vi "Using GXML For Packet Data Description.vi"() -> ()   [LabVIEW 2014]
uses:
  <vilib>/NI/GXML/_subVIs/GXML SearchParser/Search Parser.vi
  <vilib>/NI/GXML/GXML.lvlib
panel:
  out "data":T1(array[cluster])
  out "error out":errorcluster
  out "XML String Out":string
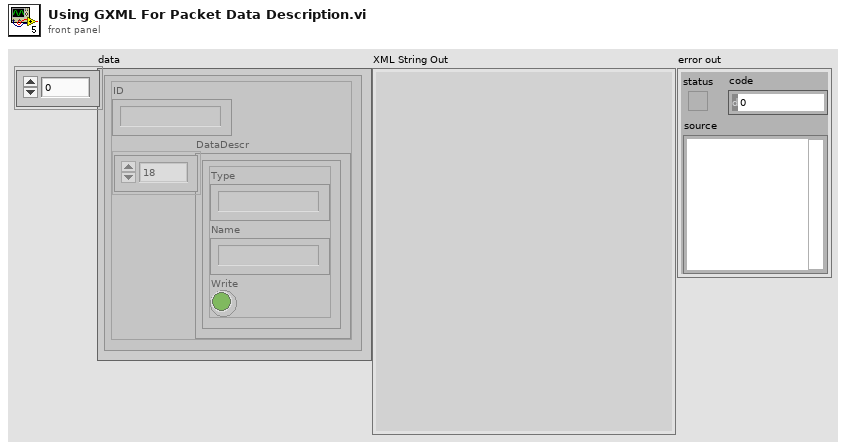
[diagram p1: front panel]
types:
  T1 = cluster{"ID":string, "DataDescr":cluster{"Type":string, "Name":string, "Write":bool}[]}[]
  T2 = cluster{"ID":string, "DataDescr":cluster{"Type":string, "Name":string, "Var":string, "Write":bool}[]}[]
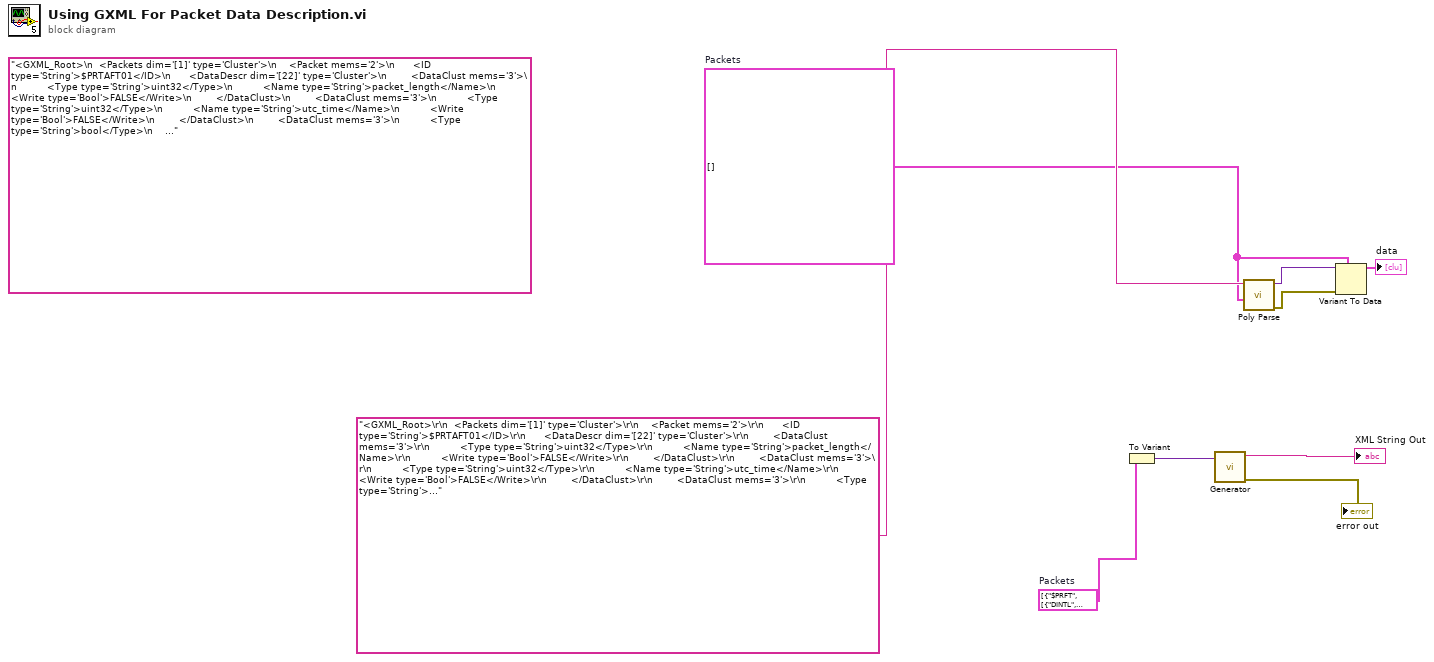
[diagram p0: block diagram]
diagram:
  w1 = T1 []  # Packets
  (unwired) "<GXML_Root>\n  <Packets dim='[1]' type='Cluster'>\n    <Packet mems='2'>\n      <ID type='String'>$PRTAFT01</ID>\n      <DataDescr dim='[22]' type='Cluster'>\n        <DataClust mems='3'>\n          <Type type='String'>uint32</Type>\n          <Name type='String'>packet_length</Name>\n          <Write type='Bool'>FALSE</Write>\n        </DataClust>\n        <DataClust mems='3'>\n          <Type type='String'>uint32</Type>\n          <Name type='String'>utc_time</Name>\n          <Write type='Bool'>FALSE</Write>\n        </DataClust>\n        <DataClust mems='3'>\n          <Type type='String'>bool</Type>\n          <Name type='String'>ptp_sync</Name>\n          <Write type='Bool'>FALSE</Write>\n        </DataClust>\n        <DataClust mems='3'>\n          <Type type='String'>uint32</Type>\n          <Name type='String'>crio_temp</Name>\n          <Write type='Bool'>FALSE</Write>\n        </DataClust>\n        <DataClust mems='3'>\n          <Type type='String'>str</Type>\n          <Name type='String'>flight_num</Name>\n          <Write type='Bool'>FALSE</Write>\n        </DataClust>\n        <DataClust mems='3'>\n          <Type type='String'>uint8</Type>\n          <Name type='String'>crio_fpga_run</Name>\n          <Write type='Bool'>FALSE</Write>\n        </DataClust>\n        <DataClust mems='3'>\n          <Type type='String'>uint8</Type>\n          <Name type='String'>crio_rtc_run</Name>\n          <Write type='Bool'>FALSE</Write>\n        </DataClust>\n        <DataClust mems='3'>\n          <Type type='String'>uint8</Type>\n          <Name type='String'>crio_status</Name>\n          <Write type='Bool'>FALSE</Write>\n        </DataClust>\n        <DataClust mems='3'>\n          <Type type='String'>uint16</Type>\n          <Name type='String'>crio_UDP_num</Name>\n          <Write type='Bool'>FALSE</Write>\n        </DataClust>\n        <DataClust mems='3'>\n          <Type type='String'>str</Type>\n          <Name type='String'>crio_mem_used</Name>\n          <Write type='Bool'>FALSE</Write>\n        </DataClust>\n        <DataClust mems='3'>\n          <Type type='String'>str</Type>\n          <Name type='String'>crio_disktype</Name>\n          <Write type='Bool'>FALSE</Write>\n        </DataClust>\n        <DataClust mems='3'>\n          <Type type='String'>str</Type>\n          <Name type='String'>crio_aux_out3</Name>\n          <Write type='Bool'>FALSE</Write>\n        </DataClust>\n        <DataClust mems='3'>\n          <Type type='String'>uint32</Type>\n          <Name type='String'>pressure_alt</Name>\n          <Write type='Bool'>FALSE</Write>\n        </DataClust>\n        <DataClust mems='3'>\n          <Type type='String'>int32</Type>\n          <Name type='String'>ind_air_speed</Name>\n          <Write type='Bool'>FALSE</Write>\n        </DataClust>\n        <DataClust mems='3'>\n          <Type type='String'>int32</Type>\n          <Name type='String'>rad_alt</Name>\n          <Write type='Bool'>FALSE</Write>\n        </DataClust>\n        <DataClust mems='3'>\n          <Type type='String'>uint8</Type>\n          <Name type='String'>unused_1</Name>\n          <Write type='Bool'>FALSE</Write>\n        </DataClust>\n        <DataClust mems='3'>\n          <Type type='String'>uint8</Type>\n          <Name type='String'>unused_2</Name>\n          <Write type='Bool'>FALSE</Write>\n        </DataClust>\n        <DataClust mems='3'>\n          <Type type='String'>uint8</Type>\n          <Name type='String'>deiced_temp_flag</Name>\n          <Write type='Bool'>FALSE</Write>\n        </DataClust>\n        <DataClust mems='3'>\n          <Type type='String'>uint8</Type>\n          <Name type='String'>wow_flag</Name>\n          <Write type='Bool'>FALSE</Write>\n        </DataClust>\n        <DataClust mems='3'>\n          <Type type='String'>uint8</Type>\n          <Name type='String'>heimann_calib_flag</Name>\n          <Write type='Bool'>FALSE</Write>\n        </DataClust>\n        <DataClust mems='3'>\n          <Type type='String'>int32</Type>\n          <Name type='String'>jci140_signal</Name>\n          <Write type='Bool'>FALSE</Write>\n        </DataClust>\n        <DataClust mems='3'>\n          <Type type='String'>int32</Type>\n          <Name type='String'>jci140_range</Name>\n          <Write type='Bool'>FALSE</Write>\n        </DataClust>\n      </DataDescr>\n    </Packet>\n  </Packets>\n</GXML_Root>\n"
  w6 = T2 [{"ID"="$PRFT", "DataDescr"=[{"Type"="DINTL", "Name"="GenericInt 1", "Var"="crd_int", "Write"=TRUE}, {"Type"="DBL", "Name"="Generic DBL", "Var"="pas_dbl", "Write"=TRUE}]}]  # Packets
  n1 = To Variant(anything=w6) -> (Variant=w9:variant)
  n2 = call <vilib>:"Generator.vi"("Variant"=w9) -> ("error out"=→"error out":errorcluster, "XML String Out"=→"XML String Out":string)  [unwired: 9 in]
  n3 = call-poly <vilib>:"Poly Parse.vi"("TypeDesc"=w1, "XML String In"="<GXML_Root>\r\n  <Packets dim='[1]' type='Cluster'>\r\n    <Packet mems='2'>\r\n      <ID type='String'>$PRTAFT01</ID>\r\n      <DataDescr dim='[22]' type='Cluster'>\r\n        <DataClust mems='3'>\r\n          <Type type='String'>uint32</Type>\r\n          <Name type='String'>packet_length</Name>\r\n          <Write type='Bool'>FALSE</Write>\r\n        </DataClust>\r\n        <DataClust mems='3'>\r\n          <Type type='String'>uint32</Type>\r\n          <Name type='String'>utc_time</Name>\r\n          <Write type='Bool'>FALSE</Write>\r\n        </DataClust>\r\n        <DataClust mems='3'>\r\n          <Type type='String'>bool</Type>\r\n          <Name type='String'>ptp_sync</Name>\r\n          <Write type='Bool'>FALSE</Write>\r\n        </DataClust>\r\n        <DataClust mems='3'>\r\n          <Type type='String'>uint32</Type>\r\n          <Name type='String'>crio_temp</Name>\r\n          <Write type='Bool'>FALSE</Write>\r\n        </DataClust>\r\n        <DataClust mems='3'>\r\n          <Type type='String'>str</Type>\r\n          <Name type='String'>flight_num</Name>\r\n          <Write type='Bool'>FALSE</Write>\r\n        </DataClust>\r\n        <DataClust mems='3'>\r\n          <Type type='String'>uint8</Type>\r\n          <Name type='String'>crio_fpga_run</Name>\r\n          <Write type='Bool'>FALSE</Write>\r\n        </DataClust>\r\n        <DataClust mems='3'>\r\n          <Type type='String'>uint8</Type>\r\n          <Name type='String'>crio_rtc_run</Name>\r\n          <Write type='Bool'>FALSE</Write>\r\n        </DataClust>\r\n        <DataClust mems='3'>\r\n          <Type type='String'>uint8</Type>\r\n          <Name type='String'>crio_status</Name>\r\n          <Write type='Bool'>FALSE</Write>\r\n        </DataClust>\r\n        <DataClust mems='3'>\r\n          <Type type='String'>uint16</Type>\r\n          <Name type='String'>crio_UDP_num</Name>\r\n          <Write type='Bool'>FALSE</Write>\r\n        </DataClust>\r\n        <DataClust mems='3'>\r\n          <Type type='String'>str</Type>\r\n          <Name type='String'>crio_mem_used</Name>\r\n          <Write type='Bool'>FALSE</Write>\r\n        </DataClust>\r\n        <DataClust mems='3'>\r\n          <Type type='String'>str</Type>\r\n          <Name type='String'>crio_disktype</Name>\r\n          <Write type='Bool'>FALSE</Write>\r\n        </DataClust>\r\n        <DataClust mems='3'>\r\n          <Type type='String'>str</Type>\r\n          <Name type='String'>crio_aux_out3</Name>\r\n          <Write type='Bool'>FALSE</Write>\r\n        </DataClust>\r\n        <DataClust mems='3'>\r\n          <Type type='String'>uint32</Type>\r\n          <Name type='String'>pressure_alt</Name>\r\n          <Write type='Bool'>FALSE</Write>\r\n        </DataClust>\r\n        <DataClust mems='3'>\r\n          <Type type='String'>int32</Type>\r\n          <Name type='String'>ind_air_speed</Name>\r\n          <Write type='Bool'>FALSE</Write>\r\n        </DataClust>\r\n        <DataClust mems='3'>\r\n          <Type type='String'>int32</Type>\r\n          <Name type='String'>rad_alt</Name>\r\n          <Write type='Bool'>FALSE</Write>\r\n        </DataClust>\r\n        <DataClust mems='3'>\r\n          <Type type='String'>uint8</Type>\r\n          <Name type='String'>unused_1</Name>\r\n          <Write type='Bool'>FALSE</Write>\r\n        </DataClust>\r\n        <DataClust mems='3'>\r\n          <Type type='String'>uint8</Type>\r\n          <Name type='String'>unused_2</Name>\r\n          <Write type='Bool'>FALSE</Write>\r\n        </DataClust>\r\n        <DataClust mems='3'>\r\n          <Type type='String'>uint8</Type>\r\n          <Name type='String'>deiced_temp_flag</Name>\r\n          <Write type='Bool'>FALSE</Write>\r\n        </DataClust>\r\n        <DataClust mems='3'>\r\n          <Type type='String'>uint8</Type>\r\n          <Name type='String'>wow_flag</Name>\r\n          <Write type='Bool'>FALSE</Write>\r\n        </DataClust>\r\n        <DataClust mems='3'>\r\n          <Type type='String'>uint8</Type>\r\n          <Name type='String'>heimann_calib_flag</Name>\r\n          <Write type='Bool'>FALSE</Write>\r\n        </DataClust>\r\n        <DataClust mems='3'>\r\n          <Type type='String'>int32</Type>\r\n          <Name type='String'>jci140_signal</Name>\r\n          <Write type='Bool'>FALSE</Write>\r\n        </DataClust>\r\n        <DataClust mems='3'>\r\n          <Type type='String'>int32</Type>\r\n          <Name type='String'>jci140_range</Name>\r\n          <Write type='Bool'>FALSE</Write>\r\n        </DataClust>\r\n      </DataDescr>\r\n    </Packet>\r\n  </Packets>\r\n</GXML_Root>\r\n") -> ("error out"=w3:errorcluster, "Parsed Data"=w5:variant)  [unwired: 8 in]
  n4 = Variant To Data(error in=w3, type=w1, Variant=w5) -> (data=→"data":T1)  [unwired: 1 out]
